vi "seconds_to_delay.vi"(11 "delay time (s)":dbl) -> ()   [LabVIEW 2015]
uses:
  global_stop_calibration.vi
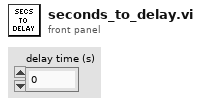
[diagram p1: front panel]
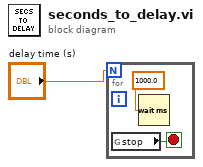
[diagram p0: block diagram]
diagram:
  n1 = for {
    N: "delay time (s)" -> [_]
    stop <- w2 stop-if-true
    n2 = global read "global_stop_calibration.vi" "stop"() -> (w2:bool)
    n3 = Wait (ms)(milliseconds to wait=1000.0 ("y")) -> ()  [unwired: 1 out]
  }
